vi "Quick Stacks.vi"(7 "Calling VI Ref":refnum<vi>) -> ()   [LabVIEW 2020]
uses:
  Hardware Configuration/Hardware Configuration Controls/Device Function.ctl
  Hardware Configuration/Hardware Configuration Controls/Device Type.ctl
  Quick Stacks Type Defs/Quick Stacks Notifier Type.ctl
  Quick Stacks Type Defs/Quick Stack Actions.ctl
  <vilib>/Utility/miscctls.llb/LVPointTypeDef.ctl
  Tools/Log File/Log File Type Defs/Log File Actions.ctl
  Device Library/Stages/Stages Controls/Stage Actions.ctl
  Device Library/Cameras/Camera Controls/Generic Camera Actions.ctl
  Color Steps/Color Steps Type Def/Color Step Actions.ctl
  Tools/TIFF Image Read and Write/ImageJ TIF Type Defs/TIF Write Image Information.ctl
  Laser Control/Laser Power Control/Laser Power Control Type Defs/Laser Power Ctrl Messenger Actions.ctl
  85f4c13c-7b78-49d2-bcfb-a940109a2fbc.vi
  Device Library/Microscopes/Polymorphic Microscope Messenger/Get Lamp State.vi
  Device Library/Microscopes/Polymorphic Microscope Messenger/Set Lamp State.vi
  shell32.dll
panel:
  out "Lamp Error":bool
  in  "Lamp":bool
  out "Current Delay Time (s)":dbl format="%.1f"
  in  "Camera 02":bool=TRUE
  in  "Camera 01":bool=TRUE
  out "Current Cycle":u16
  out "Current Step":u16
  in  "Start":bool
  in  "Number of Cycles":u16=1 min=1
  in  "Cycle Delay (s)":u32
  in  "Frames Per Step":u16=1 min=1
  in  "Base Save Path":path
  in  "File Name":string="Test Image"
  out "Z Range (µm)":dbl
  in  "Number of Steps":u16=1
  out "Step Size (µm)":dbl format="%#_3g"
  out "End Position (µm)":dbl
  out "Start Position (µm)":dbl
  in  "Set Z End":bool
  in  "Set Z Start":bool
  in  "Quit":bool
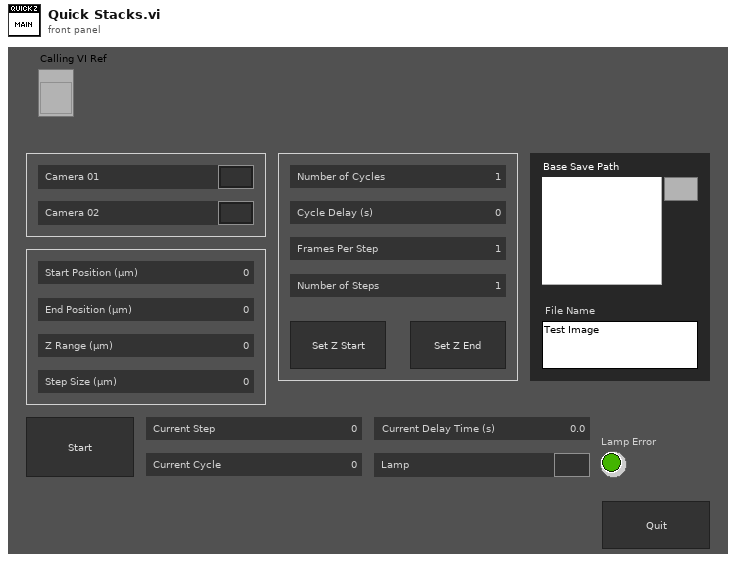
[diagram p1: front panel]
types:
  T1 = typedef "Device Function.ctl" = enum16{"Primary", "Secondary", "Overview", "Wide Field Drift Correction", "642 nm Excitation", "560 nm Excitation", "940 nm Excitation", "546 nm Excitation", "488 nm Excitation", "405 nm Excitation", "Objective Drift Correction", "4Pi Objective Lock", "Objective XY", "Objective Z", "Sample XY", "Sample Coarse Z", "Sample Z", "4Pi Lower", "4Pi Upper", "Mojo", "Adj Cavity", "Line Scanning", "Alert"}
  T2 = typedef "Device Type.ctl" = enum16{"AOTF", "Camera", "Deformable Mirror", "Laser", "Microscope Base", "Shutter", "Stage", "Waveform", "FPGA", "Email", "Filter Wheel", "Spinning Disk"}
  T3 = typedef "Log File Actions.ctl" = enum16{"Open File", "Write"}
  T4 = enum16{"Always On", "Always Off", "Off While Running"}
  T5 = typedef "LVPointTypeDef.ctl" = cluster{"Horizontal":i16, "Vertical":i16}
  T6 = typedef "Quick Stack Actions.ctl" = enum16{"Idle", "Update Range", "Start Acquisition", "Initial C Step", "Open File", "Close File", "Start Camera", "Stop Camera", "Wait New Frame", "Laser On", "Laser Off", "Get Image", "Step Z", "Move to Z Start", "Step Color", "Check Cycle", "Abort", "Exit Loop", "Quit"}
  T7 = typedef "Quick Stacks Notifier Type.ctl" = cluster{"Actions":T6, "Start Z (µm)":dbl, "End Z (µm)":dbl, "Z Size (µm)":dbl, "Num of Steps":u16, "Frames per Step":u16, "Cycle Delay (s)":u32, "Num of Cycles":u16, "Save Path":path, "Running?":bool, "Save File Refs":refnum<file>[]}
  T8 = typedef "LVRectTypeDef.ctl" = cluster{"Left":i16, "Top":i16, "Right":i16, "Bottom":i16}
  T9 = typedef "LVBoundsTypeDef.ctl" = cluster{"Width":u32, "Height":u32}
  T10 = enum8{"Enabled", "Disabled", "Disabled and Grayed Out"}
  T11 = typedef "Generic Camera Actions.ctl" = enum16{"Status", "Live Preview", "Capture", "Abort", "Set Exposure Time (s)", "Get Exposure Time (s)", "Record Settings", "Binning", "Set ROI", "Get ROI", "Defect Correction On?", "Cooler On?", "Fan On?", "Quit"}
  T12 = typedef "Stage Actions.ctl" = enum16{"Get Position", "MVR", "MOVE", "HALT", "ONTARGET", "ERROR", "REFERENCE", "INIT", "VELOCITY", "STATUS", "EXIT", "HOME", "ZEROPOS", "NANOPOS", "ANALOG", "QUIT"}
  T13 = typedef "Color Step Actions.ctl" = enum16{"Add Step", "Update Step", "Remove Step", "Clear All", "Get Status", "Next Step", "Go To Step", "Save Preset", "Change Preset", "Update Names", "Quit"}
  T14 = typedef "TIF Write Image Information.ctl" = cluster{"Image Width (Pixels)":u32, "Image Height (Pixels)":u32, "Pixel Width (µm)":dbl, "Pixel Height (µm)":dbl, "Bits Per Sample (e.g. 16)":u32, "No. of Frames":u32, "No. of Slices":u32, "Time Step (sec)":dbl, "Z Step (µm)":dbl}
  T15 = typedef "Laser Power Ctrl Messenger Actions.ctl" = enum16{"All Active On", "All Off", "Adjust Power", "Line On/Off", "Get Status"}
  T16 = typedef "IMAQ Image.ctl" = refnum<image>
  T17 = typedef "Camera IMAQ Key Info.ctl" = cluster{"Frame":u32, "Sensor Height":i32, "Sensor Width":i32, "ROI Height":i32, "ROI Width":i32, "ROI Enable?":bool, "Bit per Pixel":u8}
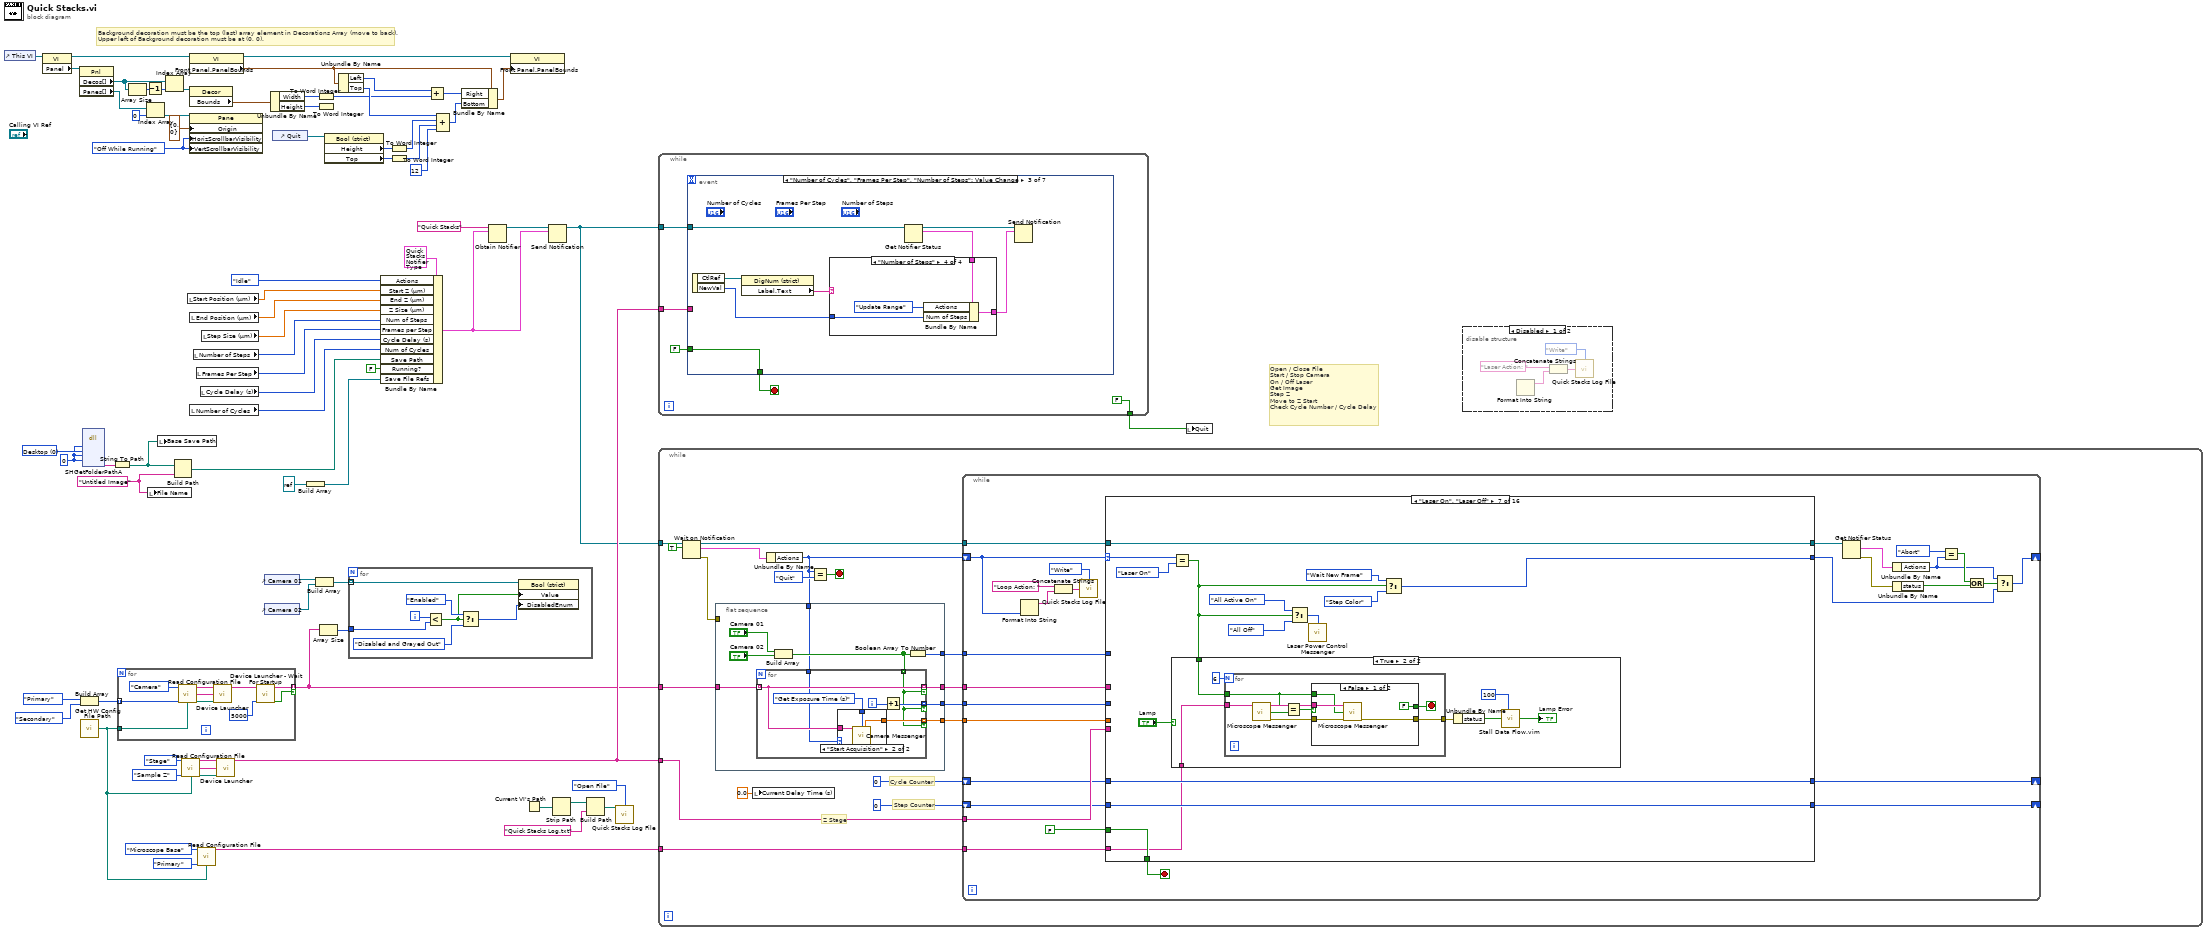
[diagram p0: block diagram]
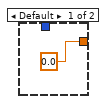
[diagram p3: hidden frame]
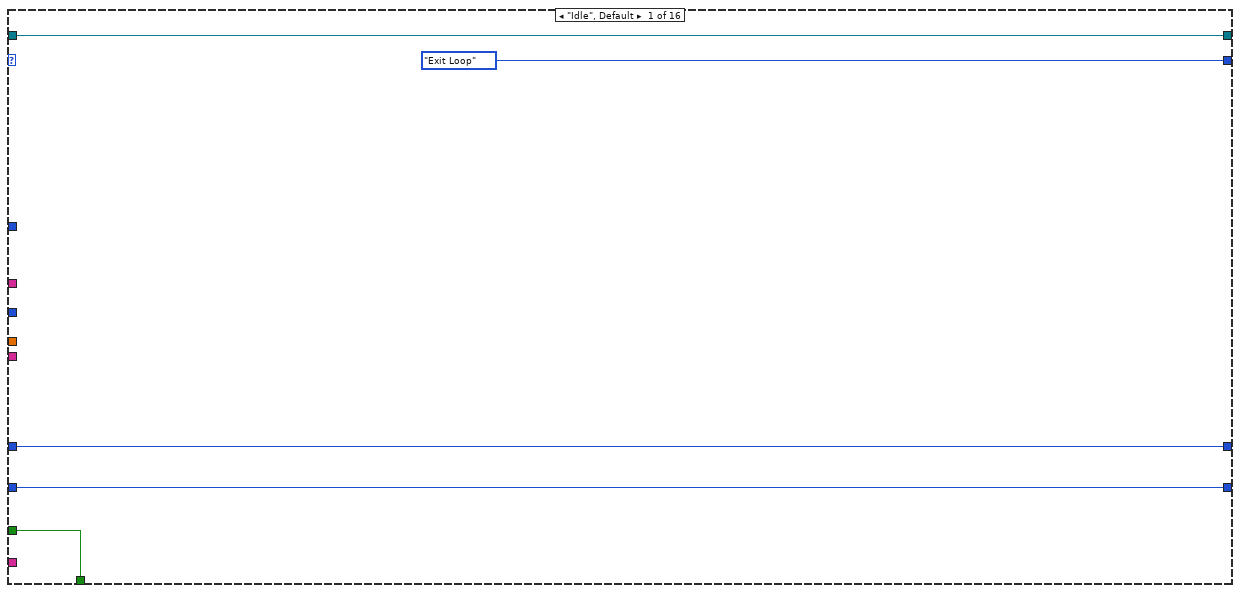
[diagram p4: hidden frame]
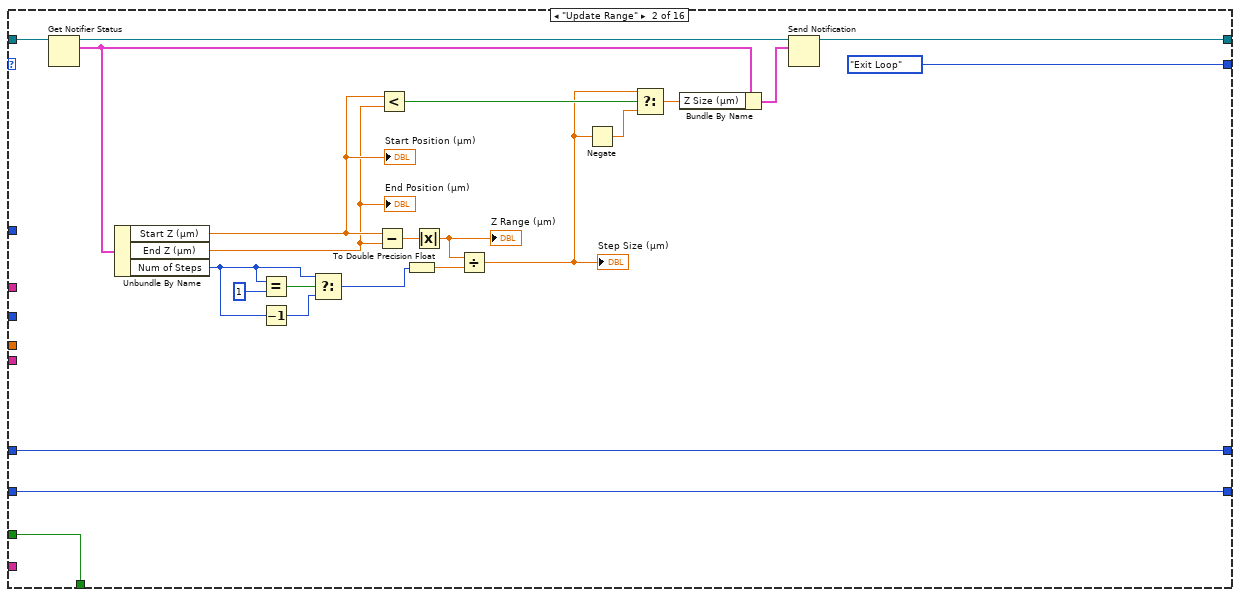
[diagram p5: hidden frame]
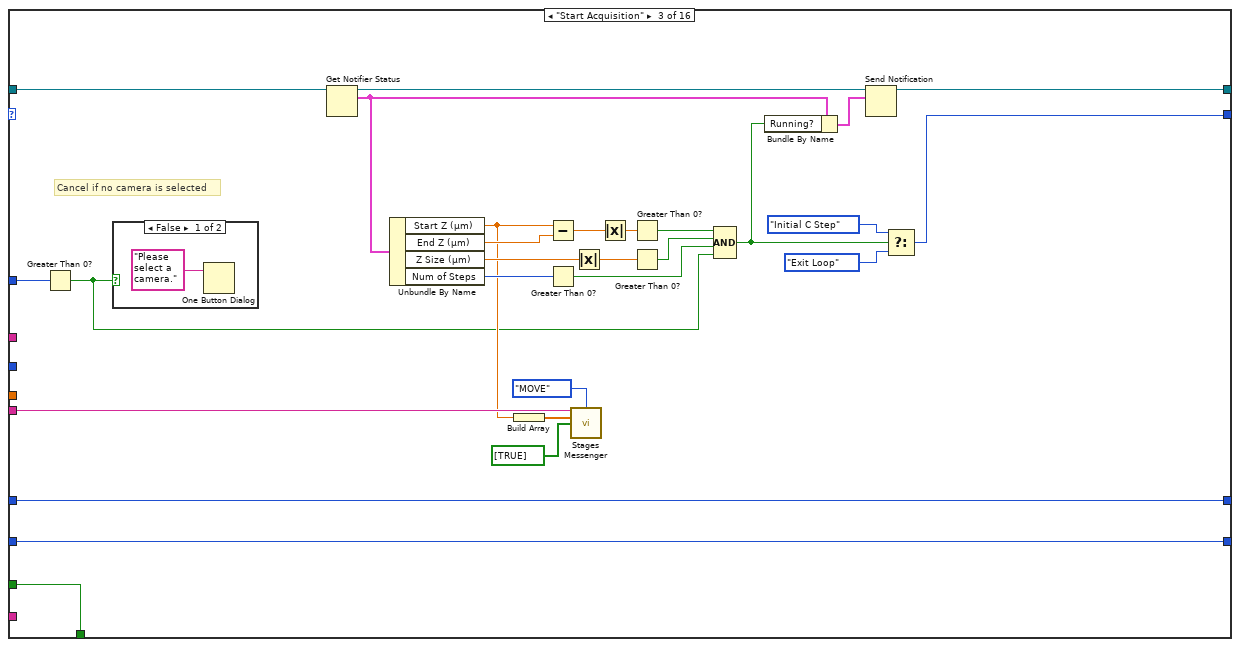
[diagram p6: hidden frame]
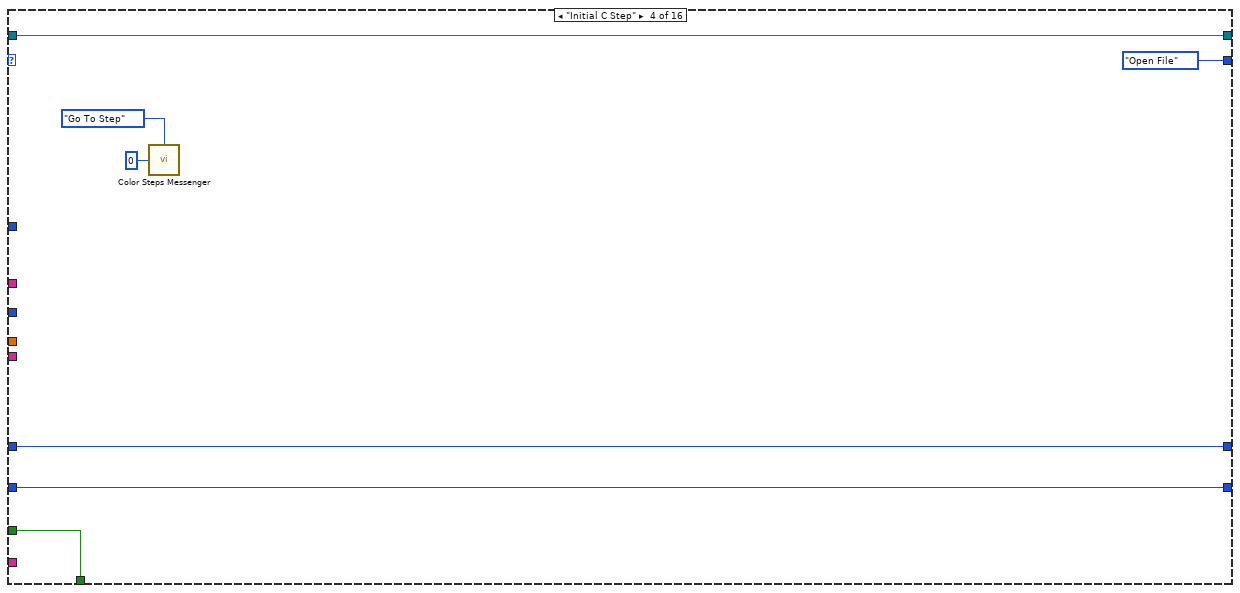
[diagram p8: hidden frame]
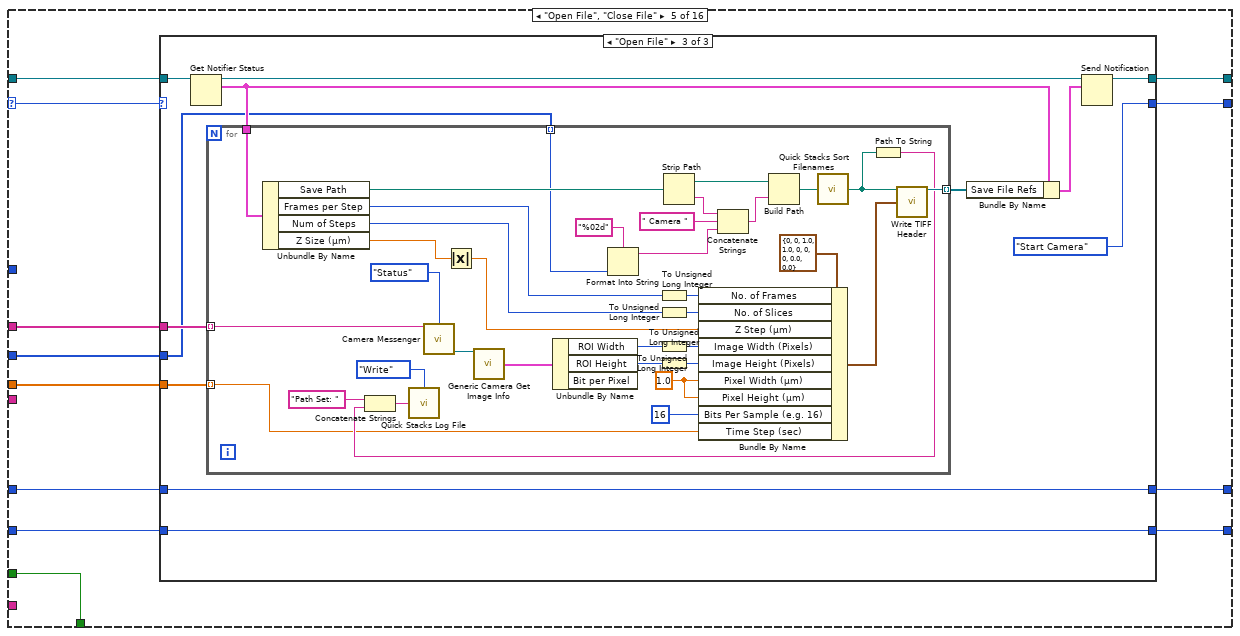
[diagram p9: hidden frame]
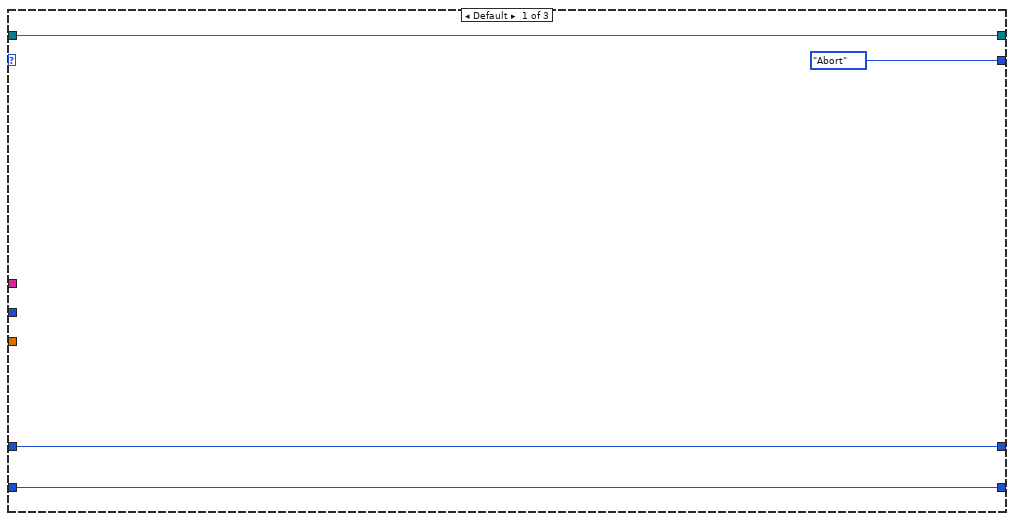
[diagram p10: hidden frame]
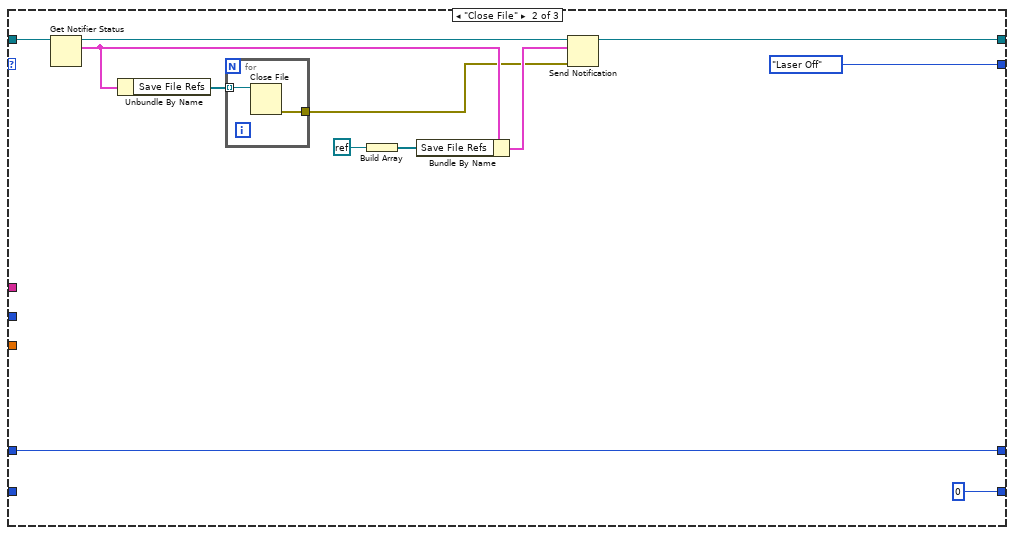
[diagram p11: hidden frame]
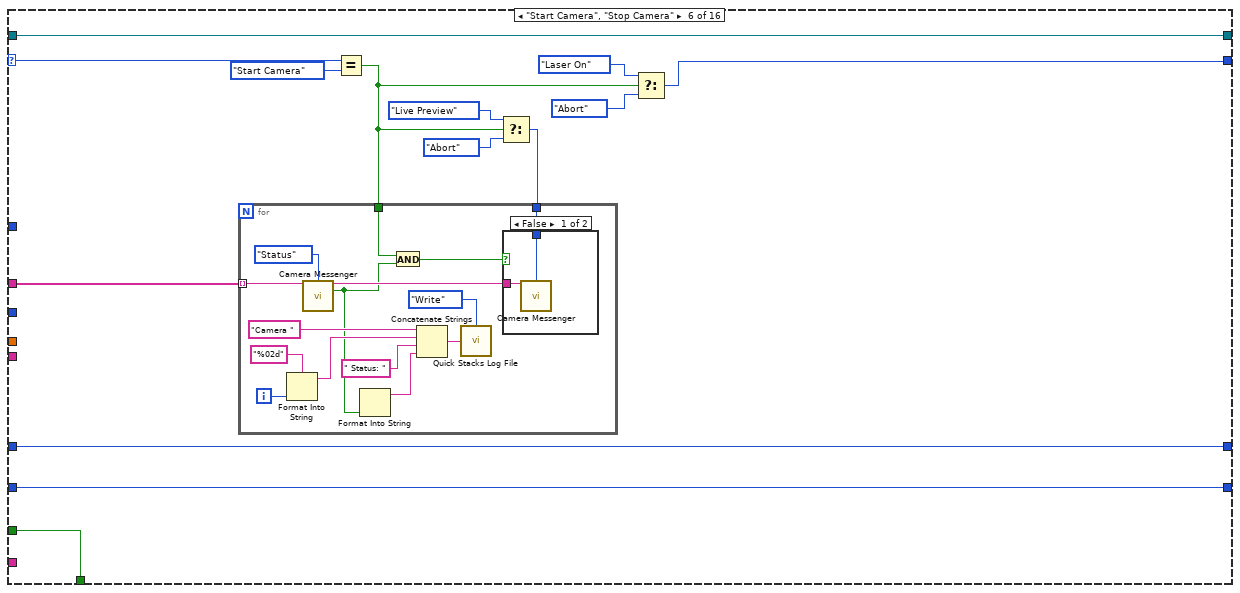
[diagram p12: hidden frame]
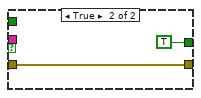
[diagram p15: hidden frame]
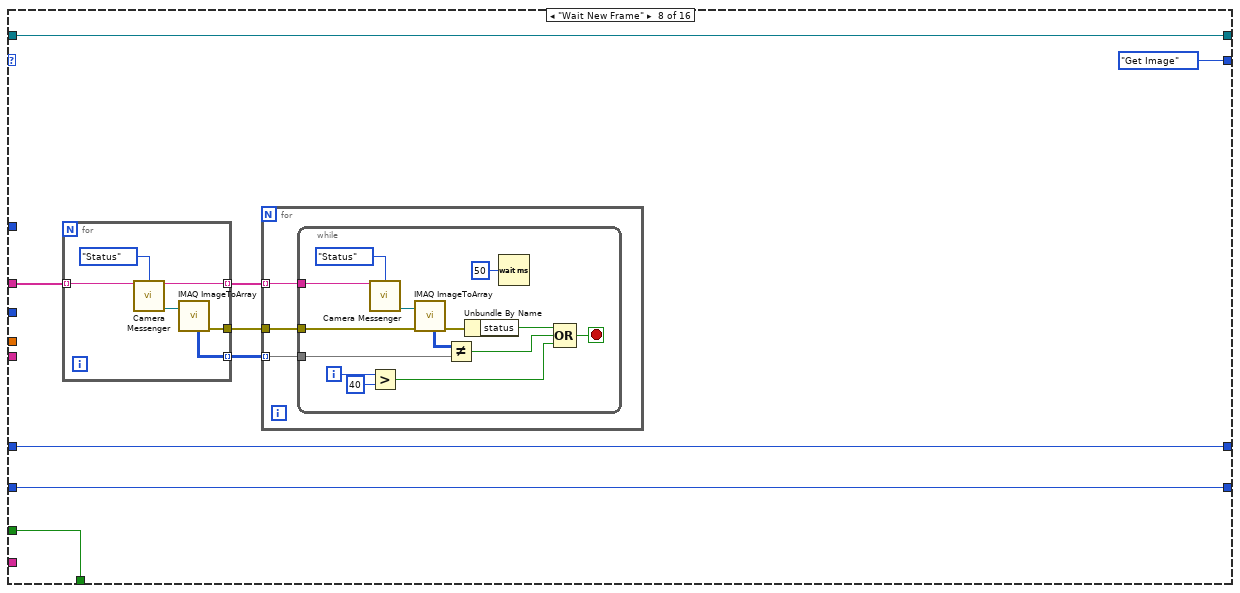
[diagram p16: hidden frame]
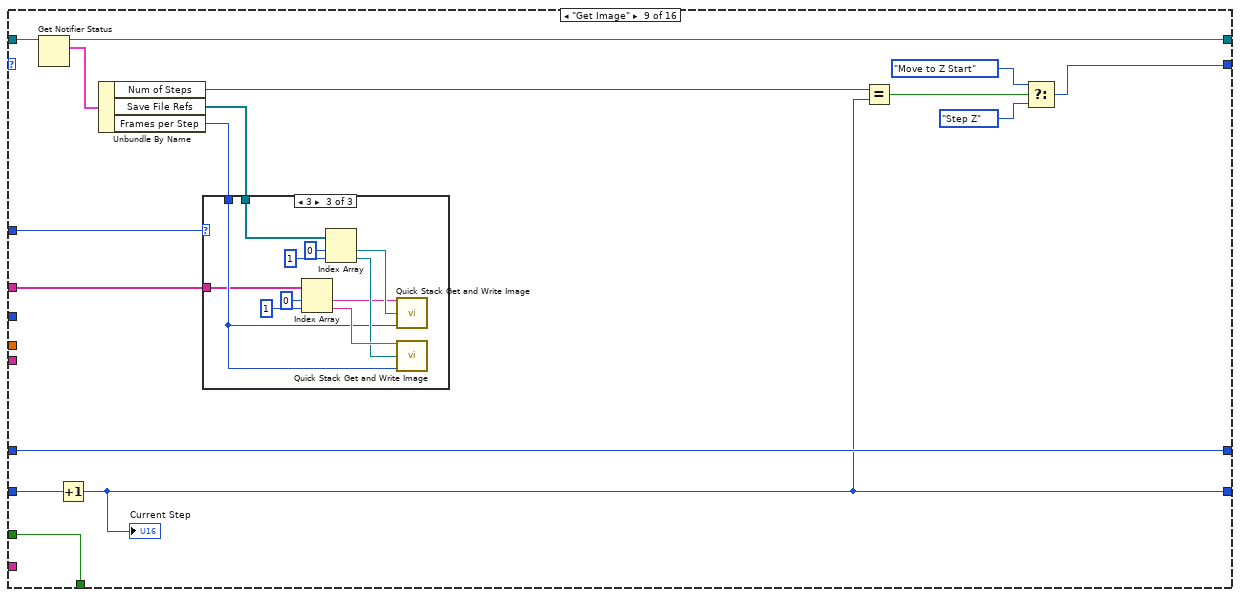
[diagram p17: hidden frame]
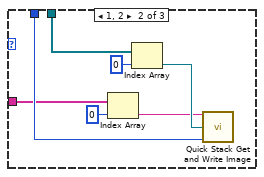
[diagram p19: hidden frame]
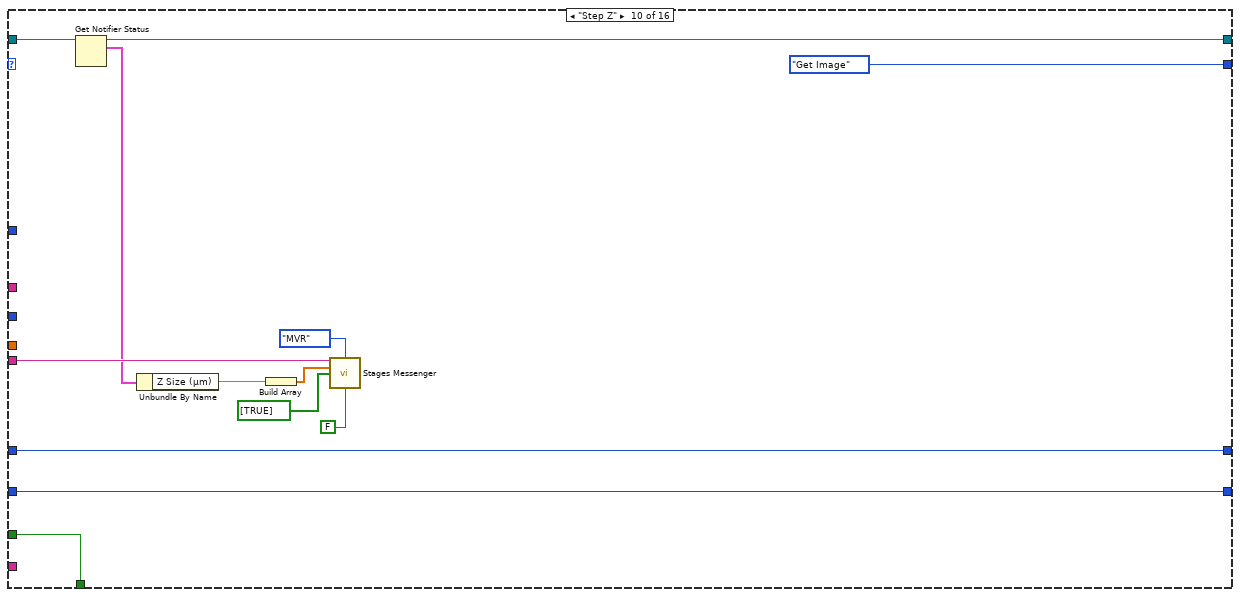
[diagram p20: hidden frame]
diagram:
  w29 = T4."Off While Running" ("Vertical Scrollbar Visibility")
  w63 = "Untitled Image"
  w66 = 0 items=["Desktop"=0, "Personal Documents"=5, "AppData"=26, "Local AppData"=28, "Common AppData"=35, "Program Files"=38, "Program Files Common"=43, "Common Documents"=46] ("Requested Path")
  w65 = 0 ("HWND")
  # "Background decoration must be the top (last) array element in Decorations Array (move to back).\nUpper left of Background decoration must be at (0, 0)."
  # "Open / Close File\nStart / Stop Camera\nOn / Off Laser\nGet Image\nStep Z\nMove to Z Start\nCheck Cycle Number / Cycle Delay"
  n1 = control-ref of="This VI"() -> (w21:refnum<vi>)
  n2 = property class="VI"(reference=w21) -> (reference out=w30:refnum<vi>, "Panel"=w22:refnum<vi>)  [unwired: 1 in, 1 out]
  n3 = property class="Pnl"(reference=w22) -> ("Decos[]"=w20:refnum<vi>[], "Panes[]"=w26:refnum<vi>[])  [unwired: 1 in, 2 out]
  n4 = Build Array(Device_Function."Primary" ("Device Function"), Device_Function."Secondary" ("Device Function")) -> (w73:T1[])
  n5 = call "Get HW Config File Path.vi"() -> ("File Path"=w2:path)  [unwired: 14 in, 1 out]
  n6 = dll-call lib="shell32.dll" fn="SHGetFolderPathA"("HWND"=w65, "nFolder"=w66, "hToken"=w65, "dwFlags"=w65) -> ("pszPath"=w64:string)  [unwired: 9 in, 2 out]
  n7 = String To Path(string=w64) -> (path=w62:path)
  n8 = for {
    tunnel: w73 -> [w81] mode=indexing
    tunnel: w2 -> [w80]
    tunnel: [w78] -> w14 mode=indexing if=w77
    n9 = call "Read Configuration File.vi"("Device Type"=Device_Type."Camera", "Device Function"=w81, "Config File Path"=w80) -> ("Unique Notifier Name"=w83:string, "Device Ports/IDs/Channels"=w85:string[], "Device Engine Path"=w84:path)  [unwired: 9 in, 1 out]
    n10 = call "Device Launcher.vi"("Notifier Name"=w83, "Device Ports/IDs/Channels"=w85, "Device Engine Path"=w84) -> ("Notifier Name"=w79:string)  [unwired: 11 in, 1 out]
    n11 = call "Device Launcher - Wait For Startup.vi"("Notifier Name"=w79, "Wait Time (ms)"=5000) -> ("Notifier Name (Dup)"=w78:string, "Running?"=w77:bool)  [unwired: 12 in]
  }
  n12 = Array Size(array=w20) -> (size(s)=w18:i32)
  n13 = Decrement(x=w18) -> (x-1=w19:i32)
  n14 = Index Array(array=w26, index=0) -> (element=w25:refnum<vi>)
  n15 = local write "File Name"(w63) -> ()
  n16 = local write "Base Save Path"(w62) -> ()
  n17 = Index Array(array=w20, index=w19) -> (element=w28:refnum<vi>)
  n18 = Build Path(base path=w62, name or relative path=w63) -> (appended path=w52:path)
  n19 = call "Read Configuration File.vi"("Device Type"=Device_Type."Stage", "Device Function"=Device_Function."Sample Z", "Config File Path"=w2) -> ("Unique Notifier Name"=w68:string, "Device Ports/IDs/Channels"=w70:string[], "Device Engine Path"=w69:path)  [unwired: 9 in, 1 out]
  n20 = local read "Start Position (µm)"() -> (w53:dbl)
  n21 = property class="VI"(reference=w30) -> (reference out=w32:refnum<vi>, "Front Panel.PanelBounds"=w33:T8)  [unwired: 1 in, 1 out]
  n22 = property class="Decor"(reference=w28) -> ("Bounds"=w31:T9)  [unwired: 1 in, 2 out]
  n23 = property class="Pane"(reference=w25, "Origin"=T5 {"Horizontal"=0, "Vertical"=0}, "HorizScrollbarVisibility"=w29, "VertScrollbarVisibility"=w29) -> ()  [unwired: 1 in, 2 out]
  n24 = local read "End Position (µm)"() -> (w54:dbl)
  n25 = local read "Number of Cycles"() -> (w59:u16)
  n26 = local read "Number of Steps"() -> (w56:u16)
  n27 = local read "Frames Per Step"() -> (w57:u16)
  n28 = call "Read Configuration File.vi"("Device Type"=Device_Type."Microscope Base", "Device Function"=Device_Function."Primary", "Config File Path"=w2) -> ("Unique Notifier Name"=w1:string)  [unwired: 9 in, 3 out]
  n29 = local read "Cycle Delay (s)"() -> (w58:u32)
  n30 = local read "Step Size (µm)"() -> (w55:dbl)
  n31 = call "Device Launcher.vi"("Notifier Name"=w68, "Device Ports/IDs/Channels"=w70, "Device Engine Path"=w69) -> ("Notifier Name"=w51:string)  [unwired: 11 in, 1 out]
  n32 = control-ref of="Camera 01"() -> (w13:refnum<vi>)
  n33 = control-ref of="Camera 02"() -> (w12:refnum<vi>)
  n34 = Unbundle By Name(w31) -> ("Width"=w36:u32, "Height"=w39:u32)
  n35 = control-ref of="Quit"() -> (w23:refnum<vi>)
  n36 = Build Array(refnum<file> refnum ("Save File Ref")) -> (w15:refnum<file>[])
  n37 = Build Array(w13, w12) -> (w11:refnum<vi>[])
  n38 = To Word Integer(number=w36) -> (16bit integer=w38:i16)
  n39 = To Word Integer(number=w39) -> ()  [unwired: 1 out]
  n40 = Array Size(array=w14) -> (size(s)=w10:i32)
  n41 = property class="Bool (strict)"(reference=w23) -> ("Height"=w41:u32, "Top"=w42:i32)  [unwired: 1 in, 2 out]
  n42 = Unbundle By Name(w33) -> ("Left"=w35:i16, "Top"=w46:i16)
  n43 = for {
    tunnel: w11 -> [w92] mode=indexing
    tunnel: w10 -> [w90]
    i -> [w91]
    n44 = Less?(x=w91, y=w90) -> (x < y?=w86:bool)
    n45 = Select(t=T10."Enabled" ("Disabled"), s=w86, f=T10."Disabled and Grayed Out" ("Disabled")) -> (s? t:f=w87:T10)
    n46 = property class="Bool (strict)"(reference=w92, "Value"=w86, "DisabledEnum"=w87) -> ()  [unwired: 1 in, 2 out]
  }
  n47 = Bundle By Name(cluster=T7 {"Actions"=enum."Idle", "Start Z (µm)"=0.0, "End Z (µm)"=0.0, "Z Size (µm)"=0.0, "Num of Steps"=0, "Frames per Step"=0, "Cycle Delay (s)"=0, "Num of Cycles"=0, "Save Path"=path "", "Running?"=FALSE, "Save File Refs"=[]} ("Stack Parameters"), "Actions"=Quick_Stack_Actions."Idle", "Start Z (µm)"=w53, "End Z (µm)"=w54, "Z Size (µm)"=w55, "Num of Steps"=w56, "Frames per Step"=w57, "Cycle Delay (s)"=w58, "Num of Cycles"=w59, "Save Path"=w52, "Running?"=FALSE ("Running"), "Save File Refs"=w15) -> (w47:T7)
  n48 = To Word Integer(number=w41) -> (16bit integer=w44:i16)
  n49 = To Word Integer(number=w42) -> (16bit integer=w45:i16)
  n50 = Add(x=w35, y=w38) -> (x+y=w37:i16)
  n51 = Compound Arithmetic op=ADD(w46, w44, w45, i16 12 ("y")) -> (w40:i16)
  n52 = Bundle By Name(cluster=w33, "Right"=w37, "Bottom"=w40) -> (w34:T8)
  n53 = Obtain Notifier(name (unnamed)="Quick Stacks", notification data type=w47) -> (notifier out=w49:refnum<notifier>)  [unwired: 2 in, 2 out]
  n54 = property class="VI"(reference=w32, "Front Panel.PanelBounds"=w34) -> ()  [unwired: 1 in, 2 out]
  n55 = Current VI's Path() -> (path=w9:path)
  n56 = Send Notification(notification=w47, notifier=w49) -> (notifier out=w48:refnum<notifier>)  [unwired: 1 in, 1 out]
  n57 = Strip Path(path=w9) -> (stripped path=w8:path)  [unwired: 1 out]
  n58 = Build Path(base path=w8, name or relative path="Quick Stacks Log.txt") -> (appended path=w6:path)
  n59 = call "Quick Stacks Log File.vi"("File Path"=w6, "Actions"=Log_File_Actions."Open File") -> ()  [unwired: 14 in]
  n60 = while {
    tunnel: w48 -> [w110]
    tunnel: w14 -> [w101]
    tunnel: w51 -> [w104]
    tunnel: w1 -> [w93]
    stop <- w107 stop-if-true
    # "Z Stage"
    # "Step Counter"
    # "Cycle Counter"
    n61 = Wait on Notification(notifier=w110, ignore previous (F)=TRUE) -> (notifier out=w106:refnum<notifier>, notification=w105:T7, error out=w97:errorcluster)  [unwired: 2 in, 1 out]
    n62 = flat-sequence {
      tunnel: w101 -> [w116]
      tunnel: [w115] -> w100
      tunnel: [w114] -> w99
      tunnel: [w113] -> w98
      tunnel: w97 -> [_]
      tunnel: [w112] -> w96
      tunnel: w95 -> [w111]
      frame #0 {
        n63 = Build Array("Camera 01", "Camera 02") -> (w119:bool[])
        n64 = for {
          tunnel: w116 -> [w124] mode=indexing
          tunnel: [w124] -> w115 mode=indexing if=w121
          tunnel: w119 -> [w121] mode=indexing
          tunnel: [w125] -> w114 mode=indexing if=w121
          tunnel: [w123] -> w112 mode=indexing if=w121
          tunnel: w111 -> [w120]
          i -> [w126]
          n65 = case shown="\"Start Acquisition\"" w120 {
            tunnel: w124 -> [_ w130]
            tunnel: [0.0 ("Current Exposure Time (s)") w129] -> w123
            tunnel: Generic_Camera_Actions."Get Exposure Time (s)" ("General Camera Actions") -> [_ w128]
            frame Default {
            }
            frame "Start Acquisition" {
              n66 = call "Camera Messenger.vi"("Notifier Name"=w130, "General Camera Actions"=w128) -> ("Current Exposure Time (s)"=w129:dbl)  [unwired: 8 in, 5 out]
            }
          }
          n67 = Increment(x=w126) -> (x+1=w125:i32)
        }
        n68 = Boolean Array To Number(Boolean array=w119) -> (number=w113:u32)
      }
    }
    n69 = local write "Current Delay Time (s)"(0.0 ("Current Delay Time (s)")) -> ()
    n70 = Unbundle By Name(w105) -> ("Actions"=w95:T6)
    n71 = Equal?(x=w95, y=Quick_Stack_Actions."Quit") -> (x = y?=w107:bool)
    n72 = while {
      tunnel: w106 -> [w158]
      shift-right: [w141] -> _
      shift-left: w95 -> [w136]
      tunnel: w104 -> [w155]
      shift-right: [w151] -> _
      shift-left: u16 0 -> [w154]
      shift-right: [w152] -> _
      shift-left: u16 0 -> [w153]
      tunnel: w100 -> [w135]
      tunnel: w99 -> [w134]
      tunnel: w98 -> [w133]
      tunnel: w96 -> [w132]
      tunnel: w93 -> [w131]
      stop <- w156 stop-if-true
      n73 = Format Into String(w136) -> (resulting string=w139:string)  [unwired: 3 in, 1 out]
      n74 = Concatenate Strings("Loop Action: ", w139) -> (w140:string)
      n75 = call "Quick Stacks Log File.vi"("Actions"=Log_File_Actions."Write", "Message"=w140) -> ()  [unwired: 14 in]
      n76 = case shown="\"Laser On\", \"Laser Off\"" w136 {
        selector: w136 -> [_ _ _ _ w232 w300 w344 _ _ _ _ _ _ _ _ _]
        tunnel: w158 -> [w161 w184 w213 w222 w233 w306 w337 w373 w413 w445 w453 w468 w492 w545 w556 w562]
        tunnel: FALSE -> [w163 w185 w214 w220 w234 w313 w345 w376 w415 w446 w455 w469 w495 w546 _ _]
        tunnel: [w163 w185 w214 w220 w234 w313 w345 w376 w415 w446 w455 w469 w495 w546 TRUE TRUE] -> w156
        tunnel: [Quick_Stack_Actions."Exit Loop" ("y") Quick_Stack_Actions."Exit Loop" ("y") w202 Quick_Stack_Actions."Open File" ("y") w231 w307 w341 Quick_Stack_Actions."Get Image" ("y") w407 Quick_Stack_Actions."Get Image" ("y") Quick_Stack_Actions."Close File" ("y") w464 w487 Quick_Stack_Actions."Exit Loop" ("y") Quick_Stack_Actions."Exit Loop" ("y") Quick_Stack_Actions."Quit" ("y")] -> w142
        tunnel: w155 -> [_ _ w199 _ _ _ _ _ _ w443 w454 _ _ w540 _ _]
        tunnel: w154 -> [w160 w170 w195 w219 w227 w305 w339 w374 w410 w442 w449 w466 w494 _ w559 w564]
        tunnel: w153 -> [w159 w169 w194 w218 w225 w304 w338 w375 w414 w441 w450 w465 _ _ w558 w563]
        tunnel: [w161 w171 w192 w222 w230 w306 w337 w373 w411 w440 w448 w468 w491 w537 w554 w562] -> w150
        tunnel: [w159 w169 w194 w218 w224 w304 w338 w375 w404 w441 w450 w465 u16 0 w539 w558 w563] -> w152
        tunnel: [w160 w170 w195 w219 w226 w305 w339 w374 w410 w442 w449 w466 w474 w539 w559 w564] -> w151
        tunnel: w135 -> [_ _ _ _ w229 w301 _ w371 w401 _ _ _ w482 w533 _ _]
        tunnel: w133 -> [_ _ w188 _ _ _ _ _ w400 _ _ _ _ _ _ _]
        tunnel: w134 -> [_ _ _ _ w228 _ _ _ _ _ _ _ _ _ _ _]
        tunnel: w132 -> [_ _ _ _ w223 _ _ _ _ _ _ _ _ _ _ _]
        tunnel: w131 -> [_ _ _ _ _ _ w331 _ _ _ _ _ _ _ _ _]
        frame "Idle", Default {
        }
        frame "Update Range" {
          n77 = Get Notifier Status(notifier=w184) -> (notifier out=w183:refnum<notifier>, current notification=w182:T7)  [unwired: 1 in, 3 out]
          n78 = Unbundle By Name(w182) -> ("Start Z (µm)"=w178:dbl, "End Z (µm)"=w177:dbl, "Num of Steps"=w180:u16)
          "Start Position (µm)" <- w178
          "End Position (µm)" <- w177
          n79 = Equal?(x=w180, y=u16 1) -> (x = y?=w165:bool)
          n80 = Decrement(x=w180) -> (x-1=w166:u16)
          n81 = Select(t=w180, s=w165, f=w166) -> (s? t:f=w167:u16)
          n82 = Subtract(x=w178, y=w177) -> (x-y=w181:dbl)
          n83 = Less?(x=w178, y=w177) -> (x < y?=w175:bool)
          n84 = To Double Precision Float(number=w167) -> (double precision float=w168:dbl)
          n85 = Absolute Value(x=w181) -> (abs(x)=w179:dbl)
          "Z Range (µm)" <- w179
          n86 = Divide(x=w179, y=w168) -> (x/y=w173:dbl)
          "Step Size (µm)" <- w173
          n87 = Negate(x=w173) -> (-x=w172:dbl)
          n88 = Select(t=w173, s=w175, f=w172) -> (s? t:f=w174:dbl)
          n89 = Bundle By Name(cluster=w182, "Z Size (µm)"=w174) -> (w176:T7)
          n90 = Send Notification(notification=w176, notifier=w183) -> (notifier out=w171:refnum<notifier>)  [unwired: 1 in, 1 out]
        }
        frame "Start Acquisition" {
          # "Cancel if no camera is selected"
          n91 = Greater Than 0?(x=w188) -> (x > 0?=w187:bool)
          n92 = case shown="False" w187 {
            frame False {
              n93 = One Button Dialog(message="Please select a camera.") -> ()  [unwired: 1 in, 1 out]
            }
            frame True {
            }
          }
          n94 = Get Notifier Status(notifier=w213) -> (notifier out=w193:refnum<notifier>, current notification=w191:T7)  [unwired: 1 in, 3 out]
          n95 = Unbundle By Name(w191) -> ("Start Z (µm)"=w198:dbl, "End Z (µm)"=w212:dbl, "Z Size (µm)"=w211:dbl, "Num of Steps"=w209:u16)
          n96 = Build Array(w198) -> (w197:dbl[])
          n97 = Subtract(x=w198, y=w212) -> (x-y=w210:dbl)
          n98 = Greater Than 0?(x=w209) -> (x > 0?=w204:bool)
          n99 = call "Stages Messenger.vi"("Stage Notifier Name"=w199, "Actions"=Stage_Actions."MOVE", "Setpoint"=w197, "Axis"=bool[] [TRUE]) -> ()  [unwired: 8 in, 4 out]
          n100 = Absolute Value(x=w211) -> (abs(x)=w207:dbl)
          n101 = Absolute Value(x=w210) -> (abs(x)=w208:dbl)
          n102 = Greater Than 0?(x=w208) -> (x > 0?=w206:bool)
          n103 = Greater Than 0?(x=w207) -> (x > 0?=w205:bool)
          n104 = Compound Arithmetic op=AND(w206, w205, w204, w187) -> (w189:bool)
          n105 = Bundle By Name(cluster=w191, "Running?"=w189) -> (w190:T7)
          n106 = Send Notification(notification=w190, notifier=w193) -> (notifier out=w192:refnum<notifier>)  [unwired: 1 in, 1 out]
          n107 = Select(t=Quick_Stack_Actions."Initial C Step", s=w189, f=Quick_Stack_Actions."Exit Loop" ("y")) -> (s? t:f=w202:T6)
        }
        frame "Initial C Step" {
          n108 = call "Color Steps Messenger.vi"("Action"=Color_Step_Actions."Go To Step", "Step"=0) -> ()  [unwired: 12 in, 2 out]
        }
        frame "Open File", "Close File" {
          n109 = case shown="\"Open File\"" w232 {
            tunnel: w233 -> [w238 w250 w264]
            tunnel: [Quick_Stack_Actions."Abort" ("y") Quick_Stack_Actions."Laser Off" ("y") Quick_Stack_Actions."Start Camera" ("y")] -> w231
            tunnel: [w238 w245 w258] -> w230
            tunnel: w229 -> [_ _ w257]
            tunnel: w228 -> [_ _ w256]
            tunnel: w227 -> [w236 w240 w255]
            tunnel: [w236 w240 w255] -> w226
            tunnel: w225 -> [w235 _ w254]
            tunnel: [w235 u16 0 w254] -> w224
            tunnel: w223 -> [_ _ w253]
            frame Default {
            }
            frame "Close File" {
              n110 = Get Notifier Status(notifier=w250) -> (notifier out=w249:refnum<notifier>, current notification=w247:T7)  [unwired: 1 in, 3 out]
              n111 = Unbundle By Name(w247) -> ("Save File Refs"=w241:refnum<file>[])
              n112 = for {
                tunnel: [w252] -> w246
                tunnel: w241 -> [w251] mode=indexing
                n113 = Close File(refnum=w251) -> (error out=w252:errorcluster)  [unwired: 1 in, 1 out]
              }
              n114 = Build Array(refnum<k0> refnum) -> (w242:refnum<k0>[])
              n115 = Bundle By Name(cluster=w247, "Save File Refs"=w242) -> (w248:T7)
              n116 = Send Notification(notification=w248, notifier=w249, error in (no error)=w246) -> (notifier out=w245:refnum<notifier>)  [unwired: 1 out]
            }
            frame "Open File" {
              n117 = Get Notifier Status(notifier=w264) -> (notifier out=w263:refnum<notifier>, current notification=w262:T7)  [unwired: 1 in, 3 out]
              n118 = for {
                tunnel: w262 -> [w287]
                tunnel: [w286] -> w260 mode=indexing
                tunnel: w257 -> [w267] mode=indexing
                tunnel: w256 -> [w277] mode=indexing
                tunnel: w253 -> [w266] mode=indexing
                w293 = 1.0 ("Pixel Width (µm)")
                n119 = Unbundle By Name(w287) -> ("Save Path"=w280:path, "Frames per Step"=w290:u16, "Num of Steps"=w289:u16, "Z Size (µm)"=w291:dbl)
                n120 = call "Camera Messenger.vi"("Notifier Name"=w267, "General Camera Actions"=Generic_Camera_Actions."Status") -> ("Image Ref"=w297:T16)  [unwired: 8 in, 5 out]
                n121 = Absolute Value(x=w291) -> (abs(x)=w288:dbl)
                n122 = call "Generic Camera Get Image Info.vi"("Image Ref"=w297) -> ("Camera Image Info"=w296:T17)  [unwired: 12 in, 2 out]
                n123 = Unbundle By Name(w296) -> ("ROI Width"=w295:i32, "ROI Height"=w294:i32)  [unwired: 1 out]
                n124 = Format Into String(format string="%02d", w277) -> (resulting string=w278:string)  [unwired: 2 in, 1 out]
                n125 = To Unsigned Long Integer(number=w290) -> (unsigned 32bit integer=w271:u32)
                n126 = To Unsigned Long Integer(number=w289) -> (unsigned 32bit integer=w270:u32)
                n127 = To Unsigned Long Integer(number=w295) -> (unsigned 32bit integer=w269:u32)
                n128 = To Unsigned Long Integer(number=w294) -> (unsigned 32bit integer=w268:u32)
                n129 = Strip Path(path=w280) -> (stripped path=w282:path, name=w281:string)
                n130 = Bundle By Name(cluster=T14 {"Image Width (Pixels)"=0, "Image Height (Pixels)"=0, "Pixel Width (µm)"=1.0, "Pixel Height (µm)"=1.0, "Bits Per Sample (e.g. 16)"=0, "No. of Frames"=0, "No. of Slices"=0, "Time Step (sec)"=0.0, "Z Step (µm)"=0.0} ("Image Info"), "No. of Frames"=w271, "No. of Slices"=w270, "Z Step (µm)"=w288, "Image Width (Pixels)"=w269, "Image Height (Pixels)"=w268, "Pixel Width (µm)"=w293, "Pixel Height (µm)"=w293, "Bits Per Sample (e.g. 16)"=u32 16 ("number"), "Time Step (sec)"=w266) -> (w298:T14)
                n131 = Concatenate Strings(w281, " Camera " ("string"), w278) -> (w283:string)
                n132 = Build Path(base path=w282, name or relative path=w283) -> (appended path=w279:path)
                n133 = call "Quick Stacks Sort Filenames.vi"("Requested File Path"=w279) -> ("Resulting File Path"=w273:path)  [unwired: 14 in]
                n134 = Path To String(path=w273) -> (string=w272:string)
                n135 = Concatenate Strings("Path Set: ", w272) -> (w276:string)
                n136 = call "Quick Stacks Log File.vi"("Actions"=Log_File_Actions."Write", "Message"=w276) -> ()  [unwired: 14 in]
                n137 = call "Write TIFF Header.vi"("File Path"=w273, "Image Info"=w298) -> ("File Ref"=w286:refnum<file>)  [unwired: 11 in, 2 out]
              }
              n138 = Bundle By Name(cluster=w262, "Save File Refs"=w260) -> (w261:T7)
              n139 = Send Notification(notification=w261, notifier=w263) -> (notifier out=w258:refnum<notifier>)  [unwired: 1 in, 1 out]
            }
          }
        }
        frame "Start Camera", "Stop Camera" {
          n140 = Equal?(x=w300, y=Quick_Stack_Actions."Start Camera") -> (x = y?=w302:bool)
          n141 = Select(t=Generic_Camera_Actions."Live Preview" ("General Camera Actions"), s=w302, f=Generic_Camera_Actions."Abort") -> (s? t:f=w309:T11)
          n142 = for {
            tunnel: w309 -> [w328]
            tunnel: w302 -> [w325]
            tunnel: w301 -> [w323] mode=indexing
            i -> [w322]
            n143 = Format Into String(format string="%02d", w322) -> (resulting string=w315:string)  [unwired: 2 in, 1 out]
            n144 = call "Camera Messenger.vi"("Notifier Name"=w323, "General Camera Actions"=Generic_Camera_Actions."Status") -> ("Notifier Name Dup"=w326:string, "Running?"=w314:bool)  [unwired: 8 in, 4 out]
            n145 = Format Into String(w314) -> (resulting string=w320:string)  [unwired: 3 in, 1 out]
            n146 = And(x=w325, y=w314) -> (x .and. y?=w324:bool)
            n147 = Concatenate Strings("Camera ", w315, " Status: " ("string"), w320) -> (w319:string)
            n148 = call "Quick Stacks Log File.vi"("Actions"=Log_File_Actions."Write", "Message"=w319) -> ()  [unwired: 14 in]
            n149 = case shown="False" w324 {
              tunnel: w328 -> [w330 _]
              tunnel: w326 -> [w329 _]
              frame False {
                n150 = call "Camera Messenger.vi"("Notifier Name"=w329, "General Camera Actions"=w330) -> ()  [unwired: 8 in, 6 out]
              }
              frame True {
              }
            }
          }
          n151 = Select(t=Quick_Stack_Actions."Laser On" ("y"), s=w302, f=Quick_Stack_Actions."Abort") -> (s? t:f=w307:T6)
        }
        frame "Laser On", "Laser Off" {
          n152 = Equal?(x=w344, y=Quick_Stack_Actions."Laser On") -> (x = y?=w333:bool)
          n153 = case shown="True" "Lamp" {
            tunnel: w333 -> [_ w351]
            tunnel: w331 -> [_ w352]
            frame False {
            }
            frame True {
              n154 = for {
                N: 6 -> [_]
                tunnel: w352 -> [w360]
                tunnel: w351 -> [w355]
                tunnel: [w354] -> w349
                stop <- w353 stop-if-true
                n155 = call-poly "Microscope Messenger.vi"("Notifier Name In"=w360) -> ("Notifier Name Out"=w357:string, "Lamp State"=w359:bool, "Error Out"=w356:errorcluster)  [unwired: 12 in]
                n156 = Equal?(x=w355, y=w359) -> (x = y?=w358:bool)
                n157 = case shown="False" w358 {
                  tunnel: w357 -> [w365 _]
                  tunnel: w356 -> [w364 w367]
                  tunnel: [w363 w367] -> w354
                  tunnel: w355 -> [w362 _]
                  tunnel: [FALSE TRUE] -> w353
                  frame False {
                    n158 = call-poly "Microscope Messenger.vi"("Notifier Name In"=w365, "Lamp State"=w362, "Error In"=w364) -> ("Error Out"=w363:errorcluster)  [unwired: 11 in, 1 out]
                  }
                  frame True {
                  }
                }
              }
              n159 = Unbundle By Name(w349) -> ("status"=w348:bool)
              n160 = call "Stall Data Flow.vim"("value in"=w348, "milliseconds to wait"=u32 100) -> ("value out"=→"Lamp Error":bool)  [unwired: 1 out]
            }
          }
          n161 = Select(t=Laser_Power_Ctrl_Messenger_Actions."All Active On" ("Power Ctrl Actions"), s=w333, f=Laser_Power_Ctrl_Messenger_Actions."All Off" ("Power Ctrl Actions")) -> (s? t:f=w334:T15)
          n162 = call "Laser Power Control Messenger.vi"("Power Ctrl Actions"=w334) -> ()  [unwired: 13 in, 2 out]
          n163 = Select(t=Quick_Stack_Actions."Wait New Frame" ("y"), s=w333, f=Quick_Stack_Actions."Step Color") -> (s? t:f=w341:T6)
        }
        frame "Wait New Frame" {
          n164 = for {
            tunnel: w371 -> [w397] mode=indexing
            tunnel: [w396] -> w369 mode=indexing
            tunnel: [w395] -> w370 mode=indexing
            tunnel: [w394] -> w368
            n165 = call "Camera Messenger.vi"("Notifier Name"=w397, "General Camera Actions"=Generic_Camera_Actions."Status") -> ("Notifier Name Dup"=w395:string, "Image Ref"=w399:T16)  [unwired: 8 in, 4 out]
            n166 = call "IMAQ ImageToArray"("Image"=w399) -> ("Image Pixels (U16)"=w396:u16[][], "error out"=w394:errorcluster)  [unwired: 3 in, 3 out]
          }
          n167 = for {
            tunnel: w370 -> [w379] mode=indexing
            tunnel: w369 -> [w378] mode=indexing
            tunnel: w368 -> [w377]
            n168 = while {
              tunnel: w379 -> [w391]
              tunnel: w378 -> [w389]
              tunnel: w377 -> [w388]
              i -> [w385]
              stop <- w380 stop-if-true
              n169 = call "Camera Messenger.vi"("Notifier Name"=w391, "General Camera Actions"=Generic_Camera_Actions."Status") -> ("Image Ref"=w392:T16)  [unwired: 8 in, 5 out]
              n170 = Greater?(x=w385, y=40) -> (0:w382:bool)
              n171 = call "IMAQ ImageToArray"("error in (no error)"=w388, "Image"=w392) -> ("Image Pixels (U16)"=w390:u16[][], "error out"=w387:errorcluster)  [unwired: 2 in, 3 out]
              n172 = Not Equal?(x=w390, y=w389) -> (x != y?=w381:bool)
              n173 = Unbundle By Name(w387) -> ("status"=w383:bool)
              n174 = Wait (ms)(milliseconds to wait=u32 50) -> ()  [unwired: 1 out]
              n175 = Compound Arithmetic op=OR(w383, w381, w382) -> (w380:bool)
            }
          }
        }
        frame "Get Image" {
          n176 = Get Notifier Status(notifier=w413) -> (notifier out=w411:refnum<notifier>, current notification=w412:T7)  [unwired: 1 in, 3 out]
          n177 = Increment(x=w414) -> (x+1=w404:u16)
          "Current Step" <- w404
          n178 = Unbundle By Name(w412) -> ("Num of Steps"=w406:u16, "Save File Refs"=w403:refnum<file>[], "Frames per Step"=w402:u16)
          n179 = case shown="3" w400 {
            tunnel: w403 -> [_ w420 w428]
            tunnel: w402 -> [_ w418 w425]
            tunnel: w401 -> [_ w417 w424]
            frame 0, Default {
            }
            frame 1, 2 {
              n180 = Index Array(array=w417, index=0) -> (element=w416:string)
              n181 = Index Array(array=w420, index=0) -> (element=w419:refnum<file>)
              n182 = call "Quick Stack Get and Write Image.vi"("Notifier Name"=w416, "Write File Ref"=w419, "Num of Frames"=w418) -> ()  [unwired: 13 in]
            }
            frame 3 {
              n183 = Index Array(array=w424, index #1=0 ("index"), index #2=1 ("index")) -> (element #1=w423:string, element #2=w431:string)
              n184 = Index Array(array=w428, index #1=0 ("index"), index #2=1 ("index")) -> (element #1=w426:refnum<file>, element #2=w427:refnum<file>)
              n185 = call "Quick Stack Get and Write Image.vi"("Notifier Name"=w423, "Write File Ref"=w426, "Num of Frames"=w425) -> ()  [unwired: 13 in]
              n186 = call "Quick Stack Get and Write Image.vi"("Notifier Name"=w431, "Write File Ref"=w427, "Num of Frames"=w425) -> ()  [unwired: 13 in]
            }
          }
          n187 = Equal?(x=w406, y=w404) -> (x = y?=w409:bool)
          n188 = Select(t=Quick_Stack_Actions."Move to Z Start", s=w409, f=Quick_Stack_Actions."Step Z" ("y")) -> (s? t:f=w407:T6)
        }
        frame "Step Z" {
          n189 = Get Notifier Status(notifier=w445) -> (notifier out=w440:refnum<notifier>, current notification=w437:T7)  [unwired: 1 in, 3 out]
          n190 = Unbundle By Name(w437) -> ("Z Size (µm)"=w438:dbl)
          n191 = Build Array(w438) -> (w436:dbl[])
          n192 = call "Stages Messenger.vi"("Stage Notifier Name"=w443, "Actions"=Stage_Actions."MVR", "Setpoint"=w436, "Axis"=bool[] [TRUE], "Exit While Busy?"=FALSE) -> ()  [unwired: 7 in, 4 out]
        }
        frame "Move to Z Start" {
          n193 = Get Notifier Status(notifier=w453) -> (notifier out=w448:refnum<notifier>, current notification=w452:T7)  [unwired: 1 in, 3 out]
          n194 = Unbundle By Name(w452) -> ("Start Z (µm)"=w451:dbl)
          n195 = Build Array(w451) -> (w456:dbl[])
          n196 = call "Stages Messenger.vi"("Stage Notifier Name"=w454, "Actions"=Stage_Actions."MOVE", "Setpoint"=w456, "Axis"=bool[] [TRUE]) -> ()  [unwired: 8 in, 4 out]
        }
        frame "Step Color" {
          n197 = call "Color Steps Messenger.vi"("Action"=Color_Step_Actions."Get Status") -> ("Last Step"=w459:bool)  [unwired: 13 in, 1 out]
          n198 = case shown="True" w459 {
            tunnel: [Quick_Stack_Actions."Open File" ("y") Quick_Stack_Actions."Check Cycle" ("y")] -> w464
            frame False {
              n199 = call "Color Steps Messenger.vi"("Action"=Color_Step_Actions."Next Step") -> ()  [unwired: 13 in, 2 out]
            }
            frame True {
            }
          }
          n200 = Format Into String(w459) -> (resulting string=w462:string)  [unwired: 3 in, 1 out]
          n201 = Concatenate Strings("Last Color Step: ", w462) -> (w463:string)
          n202 = call "Quick Stacks Log File.vi"("Actions"=Log_File_Actions."Write", "Message"=w463) -> ()  [unwired: 14 in]
        }
        frame "Check Cycle" {
          n203 = Get Notifier Status(notifier=w492) -> (notifier out=w491:refnum<notifier>, current notification=w493:T7)  [unwired: 1 in, 3 out]
          n204 = Increment(x=w494) -> (x+1=w474:u16)
          "Current Cycle" <- w474
          n205 = Unbundle By Name(w493) -> ("Num of Cycles"=w473:u16, "Cycle Delay (s)"=w485:u32)
          n206 = Greater?(x=w485, y=u32 20) -> (0:w483:bool)
          n207 = To Long Integer(number=w485) -> (32bit integer=w476:i32)
          n208 = Greater Or Equal?(x=w474, y=w473) -> (x >= y?=w490:bool)
          n209 = Multiply(x=w476, y=10) -> (x*y=w475:i32)
          n210 = case shown="False" w490 {
            tunnel: w483 -> [w498 _]
            tunnel: w482 -> [w497 w528]
            tunnel: w475 -> [w496 _]
            frame False {
              n211 = case shown="True" w498 {
                tunnel: w497 -> [_ w508]
                tunnel: w496 -> [w499 w506]
                frame False {
                  n212 = for {
                    N: w499 -> [_]
                    i -> [w504]
                    n213 = Increment(x=w504) -> (x+1=w500:i32)
                    n214 = Wait (ms)(milliseconds to wait=u32 100) -> ()  [unwired: 1 out]
                    n215 = To Double Precision Float(number=w500) -> (double precision float=w503:dbl)
                    n216 = Divide(x=w503, y=10.0) -> (x/y=→"Current Delay Time (s)":dbl)
                  }
                }
                frame True {
                  n217 = flat-sequence {
                    tunnel: [w512] -> w509
                    tunnel: w508 -> [w513]
                    tunnel: [w511] -> w507
                    tunnel: w506 -> [w511]
                    tunnel: [w517] -> w510
                    tunnel: w509 -> [w517]
                    tunnel: w507 -> [w518]
                    tunnel: w510 -> [w525]
                    frame #0 {
                      n218 = for {
                        tunnel: w513 -> [w515] mode=indexing
                        tunnel: [w514] -> w512 mode=indexing
                        n219 = call "Camera Messenger.vi"("Notifier Name"=w515, "General Camera Actions"=Generic_Camera_Actions."Abort") -> ("Notifier Name Dup"=w514:string)  [unwired: 8 in, 5 out]
                      }
                    }
                    frame #1 {
                      n220 = for {
                        N: w518 -> [_]
                        i -> [w519]
                        n221 = Increment(x=w519) -> (x+1=w520:i32)
                        n222 = To Double Precision Float(number=w520) -> (double precision float=w523:dbl)
                        n223 = Divide(x=w523, y=10.0) -> (x/y=w521:dbl)
                        n224 = Wait (ms)(milliseconds to wait=u32 100) -> ()  [unwired: 1 out]
                        n225 = local write "Current Delay Time (s)"(w521) -> ()
                      }
                    }
                    frame #2 {
                      n226 = for {
                        tunnel: w525 -> [w526] mode=indexing
                        n227 = call "Camera Messenger.vi"("Notifier Name"=w526, "General Camera Actions"=Generic_Camera_Actions."Live Preview") -> ()  [unwired: 8 in, 6 out]
                      }
                    }
                  }
                }
              }
            }
            frame True {
              n228 = for {
                tunnel: w528 -> [w529] mode=indexing
                n229 = call "Camera Messenger.vi"("Notifier Name"=w529, "General Camera Actions"=Generic_Camera_Actions."Abort") -> ()  [unwired: 8 in, 6 out]
              }
            }
          }
          n230 = Format Into String(w474) -> (resulting string=w480:string)  [unwired: 3 in, 1 out]
          n231 = Concatenate Strings("Current Cycle: ", w480) -> (w481:string)
          n232 = call "Quick Stacks Log File.vi"("Actions"=Log_File_Actions."Write", "Message"=w481) -> ()  [unwired: 14 in]
          n233 = Select(t=Quick_Stack_Actions."Exit Loop", s=w490, f=Quick_Stack_Actions."Initial C Step" ("y")) -> (s? t:f=w487:T6)
        }
        frame "Abort" {
          w539 = u16 0
          n234 = for {
            tunnel: w533 -> [w549] mode=indexing
            n235 = call "Camera Messenger.vi"("Notifier Name"=w549, "General Camera Actions"=Generic_Camera_Actions."Abort") -> ()  [unwired: 8 in, 6 out]
          }
          n236 = Get Notifier Status(notifier=w545) -> (notifier out=w538:refnum<notifier>, current notification=w536:T7)  [unwired: 1 in, 3 out]
          n237 = Unbundle By Name(w536) -> ("Save File Refs"=w532:refnum<file>[], "Start Z (µm)"=w541:dbl)
          n238 = call "Laser Power Control Messenger.vi"("Power Ctrl Actions"=Laser_Power_Ctrl_Messenger_Actions."All Off") -> ()  [unwired: 13 in, 2 out]
          n239 = Bundle By Name(cluster=w536, "Actions"=Quick_Stack_Actions."Exit Loop") -> (w534:T7)
          n240 = Build Array(w541) -> (w542:dbl[])
          n241 = for {
            tunnel: w532 -> [w548] mode=indexing
            n242 = Close File(refnum=w548) -> ()  [unwired: 1 in, 2 out]
          }
          n243 = call "Stages Messenger.vi"("Stage Notifier Name"=w540, "Actions"=Stage_Actions."MOVE", "Setpoint"=w542, "Axis"=bool[] [TRUE]) -> ()  [unwired: 8 in, 4 out]
          n244 = Send Notification(notification=w534, notifier=w538) -> (notifier out=w537:refnum<notifier>)  [unwired: 1 in, 1 out]
        }
        frame "Exit Loop" {
          n245 = Get Notifier Status(notifier=w556) -> (notifier out=w555:refnum<notifier>, current notification=w553:T7)  [unwired: 1 in, 3 out]
          n246 = Bundle By Name(cluster=w553, "Running?"=FALSE ("Running")) -> (w551:T7)
          n247 = local write "Start"(FALSE ("Start")) -> ()
          n248 = Send Notification(notification=w551, notifier=w555) -> (notifier out=w554:refnum<notifier>)  [unwired: 1 in, 1 out]
        }
        frame "Quit" {
          n249 = Release Notifier(notifier=w562) -> ()  [unwired: 2 in, 3 out]
        }
      }
      n250 = Get Notifier Status(notifier=w150) -> (current notification=w149:T7, error out=w148:errorcluster)  [unwired: 1 in, 3 out]
      n251 = Unbundle By Name(w149) -> ("Actions"=w143:T6)
      n252 = Unbundle By Name(w148) -> ("status"=w146:bool)
      n253 = Equal?(x=Quick_Stack_Actions."Abort", y=w143) -> (x = y?=w145:bool)
      n254 = Or(x=w145, y=w146) -> (x .or. y?=w144:bool)
      n255 = Select(t=w143, s=w144, f=w142) -> (s? t:f=w141:T6)
    }
  }
  n256 = while {
    tunnel: w48 -> [w569]
    tunnel: w51 -> [w568]
    tunnel: [FALSE] -> w50
    stop <- w571 stop-if-true
    n257 = event shown="[2] \"Number of Cycles\", \"Frames Per Step\", \"Number of Steps\": Value Change" {
      selector: _ -> [_ _ _ _ _ _ _]
      dyn-events: _ -> [_ _ _ _ _ _ _]
      timeout: _ -> [_ _ _ _ _ _ _]
      tunnel: [w572 w584 w603 w625 w634 w643 w649] -> w571
      tunnel: FALSE -> [w572 w584 w603 w625 w634 w643 _]
      tunnel: w569 -> [_ w581 w600 w623 w632 w639 w648]
      tunnel: w568 -> [_ w580 _ _ _ _ _]
      event Timeout {
        n258 = event-data() -> ()  [unwired: 1 in, 3 out]
      }
      event "Set Z Start", "Set Z End": Value Change {
        n259 = event-data() -> ("CtlRef"=w583:refnum<vi>)  [unwired: 1 in]
        n260 = property class="Bool"(reference=w583) -> ("Label.Text"=w582:string)  [unwired: 1 in, 2 out]
        n261 = call "Stages Messenger.vi"("Stage Notifier Name"=w580, "Actions"=Stage_Actions."Get Position") -> ("Positions"=w578:dbl[])  [unwired: 10 in, 3 out]
        n262 = Index Array(array=w578, index=0) -> (element=w576:dbl)
        n263 = Get Notifier Status(notifier=w581) -> (notifier out=w575:refnum<notifier>, current notification=w574:T7)  [unwired: 1 in, 3 out]
        n264 = case shown="\"Set Z Start\"" w582 {
          tunnel: w576 -> [_ w590 w594]
          tunnel: w574 -> [w587 w591 w595]
          tunnel: [w585 w588 w592] -> w573
          frame Default {
            n265 = Bundle By Name(cluster=w587, "Actions"=Quick_Stack_Actions."Idle") -> (w585:T7)
          }
          frame "Set Z Start" {
            n266 = Bundle By Name(cluster=w591, "Actions"=Quick_Stack_Actions."Update Range", "Start Z (µm)"=w590) -> (w588:T7)
          }
          frame "Set Z End" {
            n267 = Bundle By Name(cluster=w595, "Actions"=Quick_Stack_Actions."Update Range", "End Z (µm)"=w594) -> (w592:T7)
          }
        }
        n268 = Send Notification(notification=w573, notifier=w575) -> ()  [unwired: 1 in, 2 out]
      }
      event "Number of Cycles", "Frames Per Step", "Number of Steps": Value Change {
        n269 = event-data() -> ("CtlRef"=w602:refnum<vi>, "NewVal"=w597:u16)  [unwired: 1 in]
        n270 = property class="DigNum (strict)"(reference=w602) -> ("Label.Text"=w599:string)  [unwired: 1 in, 2 out]
        n271 = Get Notifier Status(notifier=w600) -> (notifier out=w601:refnum<notifier>, current notification=w598:T7)  [unwired: 1 in, 3 out]
        n272 = case shown="\"Number of Steps\"" w599 {
          tunnel: w598 -> [w606 w610 w614 w618]
          tunnel: w597 -> [_ w608 w612 w616]
          tunnel: [w604 w607 w611 w615] -> w596
          frame Default {
            n273 = Bundle By Name(cluster=w606, "Actions"=Quick_Stack_Actions."Idle") -> (w604:T7)
          }
          frame "Number of Cycles" {
            n274 = Bundle By Name(cluster=w610, "Actions"=Quick_Stack_Actions."Idle", "Num of Cycles"=w608) -> (w607:T7)
          }
          frame "Frames Per Step" {
            n275 = Bundle By Name(cluster=w614, "Actions"=Quick_Stack_Actions."Idle", "Frames per Step"=w612) -> (w611:T7)
          }
          frame "Number of Steps" {
            n276 = Bundle By Name(cluster=w618, "Actions"=Quick_Stack_Actions."Update Range", "Num of Steps"=w616) -> (w615:T7)
          }
        }
        n277 = Send Notification(notification=w596, notifier=w601) -> ()  [unwired: 1 in, 2 out]
      }
      event "Cycle Delay (s)": Value Change {
        n278 = event-data() -> ("NewVal"=w621:u32)  [unwired: 1 in]
        n279 = Get Notifier Status(notifier=w623) -> (notifier out=w624:refnum<notifier>, current notification=w622:T7)  [unwired: 1 in, 3 out]
        n280 = Bundle By Name(cluster=w622, "Actions"=Quick_Stack_Actions."Idle", "Cycle Delay (s)"=w621) -> (w620:T7)
        n281 = Send Notification(notification=w620, notifier=w624) -> ()  [unwired: 1 in, 2 out]
      }
      event "Base Save Path", "File Name": Value Change {
        n282 = event-data() -> ()  [unwired: 1 in, 1 out]
        n283 = Build Path(base path="Base Save Path", name or relative path="File Name") -> (appended path=w626:path)
        n284 = Get Notifier Status(notifier=w632) -> (notifier out=w633:refnum<notifier>, current notification=w631:T7)  [unwired: 1 in, 3 out]
        n285 = Bundle By Name(cluster=w631, "Actions"=Quick_Stack_Actions."Idle", "Save Path"=w626) -> (w630:T7)
        n286 = Send Notification(notification=w630, notifier=w633) -> ()  [unwired: 1 in, 2 out]
      }
      event "Start": Value Change {
        n287 = event-data() -> ("NewVal"=w638:bool)  [unwired: 1 in]
        n288 = Select(t=Quick_Stack_Actions."Start Acquisition" ("Actions"), s=w638, f=Quick_Stack_Actions."Abort" ("Actions")) -> (s? t:f=w635:T6)
        n289 = Get Notifier Status(notifier=w639) -> (notifier out=w642:refnum<notifier>, current notification=w641:T7)  [unwired: 1 in, 3 out]
        n290 = Bundle By Name(cluster=w641, "Actions"=w635) -> (w640:T7)
        n291 = Send Notification(notification=w640, notifier=w642) -> ()  [unwired: 1 in, 2 out]
      }
      event "Quit": Value Change {
        n292 = event-data() -> ("NewVal"=w649:bool)  [unwired: 1 in]
        n293 = Get Notifier Status(notifier=w648) -> (notifier out=w645:refnum<notifier>, current notification=w647:T7)  [unwired: 1 in, 3 out]
        n294 = Bundle By Name(cluster=w647, "Actions"=Quick_Stack_Actions."Quit") -> (w644:T7)
        n295 = Send Notification(notification=w644, notifier=w645) -> ()  [unwired: 1 in, 2 out]
      }
    }
  }
  n296 = local write "Quit"(w50) -> ()
  n297 = disable-structure shown="Disabled" {
    frame Disabled {
      n298 = Format Into String() -> (resulting string=w651:string)  [unwired: 4 in, 1 out]
      n299 = Concatenate Strings("Laser Action: ", w651) -> (w650:string)
      n300 = call "Quick Stacks Log File.vi"("Actions"=Log_File_Actions."Write", "Message"=w650) -> ()  [unwired: 14 in]
    }
    frame Enabled {
    }
  }
